vi "Get Version.vi"(11 "PN532 COM Port":refnum<visa-resource-name>) -> (0 "error out":errorcluster, 2 "Version Data":string, 3 "PN532 COM Port":refnum<visa-resource-name>)   [LabVIEW 2012, in "NFC Driver.lvlib"]
doc: "This VI reads the 4 pages starting on the one specified by \"Address\"; i.e. If \"Address\" is 0x00 then \"16-byte data\" will return the data in pages 0x00, 0x01, 0x02 and 0x03.\n\nIt is possible to specify to get a subset of the information stored in the returned pages by using \"offset (max. 16) and \"length (max. 16)\". The desired subset of information will be returned in \"Selected substring (HEX)\" (raw hex format) and \"Selected substring (ASCII)\" (ASCII format)."
uses:
  NFC Driver.lvlib
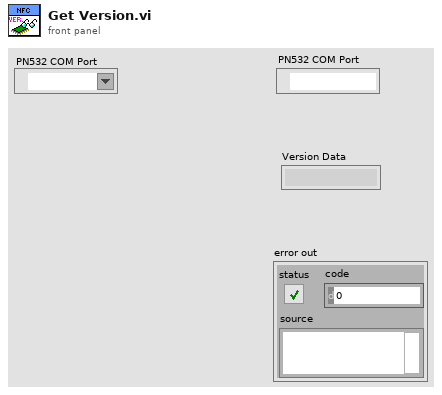
[diagram p1: front panel]
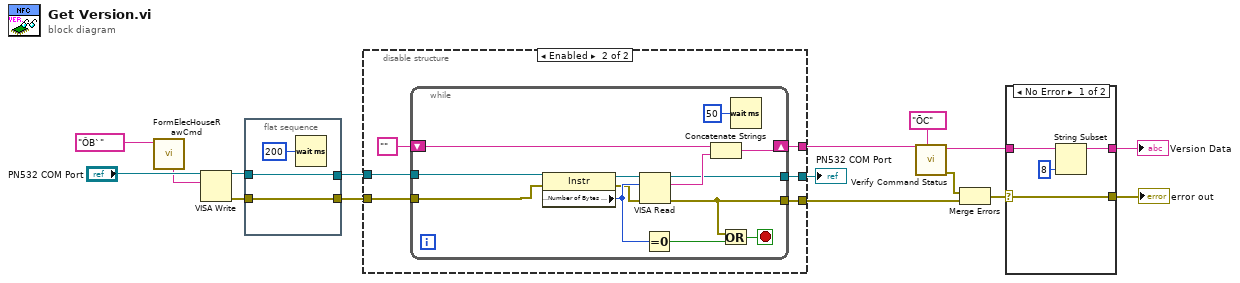
[diagram p0: block diagram]
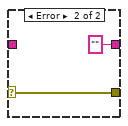
[diagram p2: hidden frame]
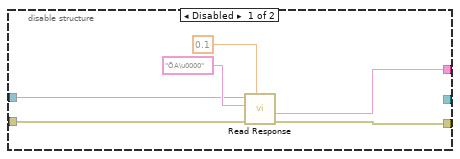
[diagram p3: hidden frame]
diagram:
  n1 = call "FormElecHouseRawCmd.vi"("Command"="ÔB`" ("string")) -> ("concatenated Cmd"=w15:string)  [unwired: 10 in]
  n2 = VISA Write(VISA resource name="PN532 COM Port", write buffer=w15) -> (VISA resource name out=w14:refnum<visa-resource-name>, error out=w12:errorcluster)  [unwired: 1 in, 1 out]
  n3 = flat-sequence {
    tunnel: w14 -> [w18]
    tunnel: [w18] -> w13
    tunnel: w12 -> [w17]
    tunnel: [w17] -> w11
    frame #0 {
      n4 = Wait (ms)(milliseconds to wait=u32 200) -> ()  [unwired: 1 out]
    }
  }
  n5 = disable-structure shown="Enabled" {
    disable-tunnel: w13 -> [w23 w31]
    disable-tunnel: w11 -> [w22 w30]
    disable-tunnel: [w21 w27] -> w10
    disable-tunnel: [w20 w29] -> w8
    disable-tunnel: [_ w26] -> w1
    frame Disabled {
      n6 = call "Read Response.vi"("Timeout (s)"=0.1, "error in (no error)"=w22, "regular expression"="ÕA\u0000", "PN532 COM Port"=w23) -> ("error out"=w21:errorcluster, "Response Data"=w20:string)  [unwired: 4 in, 2 out]
    }
    frame Enabled {
      n7 = while {
        tunnel: w31 -> [w35]
        tunnel: w30 -> [w34]
        shift-right: [w40] -> w29
        shift-left: "" -> [w42]
        tunnel: [w36] -> w27
        tunnel: [w33] -> w26
        stop <- w37 stop-if-true
        n8 = property class="Instr"(reference=w35, error in=w34) -> (reference out=w44:refnum<visa-resource-name>, error out=w39:errorcluster, "Serial Settings:Number of Bytes at Serial Port"=w43:u32)
        n9 = VISA Read(VISA resource name=w44, byte count=w43, error in (no error)=w39) -> (VISA resource name out=w33:refnum<visa-resource-name>, read buffer=w41:string, error out=w36:errorcluster)  [unwired: 1 out]
        n10 = Equal To 0?(x=w43) -> (x = 0?=w38:bool)
        n11 = Concatenate Strings(w42, w41) -> (w40:string)
        n12 = Or(x=w36, y=w38) -> (x .or. y?=w37:bool)
        n13 = Wait (ms)(milliseconds to wait=u32 50) -> ()  [unwired: 1 out]
      }
    }
  }
  "PN532 COM Port" <- w1
  n14 = call "Verify Command Status.vi"("Response Token"="ÕC", "Response"=w8) -> ("error out"=w2:errorcluster, "Data"=w3:string)  [unwired: 8 in]
  n15 = Merge Errors(w2, w10) -> (w4:errorcluster)
  n16 = case shown="No Error" w4 {
    selector: w4 -> [w48 w50]
    tunnel: [w48 w50] -> w7
    tunnel: w3 -> [w47 _]
    tunnel: [w46 "" ("Data")] -> w6
    frame No Error {
      n17 = String Subset(string=w47, length (rest)=8 ("length (rest)")) -> (substring=w46:string)  [unwired: 1 in]
    }
    frame Error {
    }
  }
  "error out" <- w7
  "Version Data" <- w6
